vi "set ChildNode.vi"(8 "error in (no error)":errorcluster caption="错误输入（无错误）", 9 "ChildNode*":refnum<data-value>, 10 "index":i32 caption="L/R", 11 "PanelLinkNode输入":refnum<class "PanelLinkNode.lvclass">) -> (0 "error out":errorcluster caption="错误输出", 3 "PanelLinkNode输出":refnum<class "PanelLinkNode.lvclass">)   [LabVIEW 2016, in "PanelLinkNode.lvclass"]
uses:
  PanelLinkNode.lvclass
  PanelObject/PanelObject.lvclass
  PanelLinkNode.lvclass/PanelLinkNode.ctl
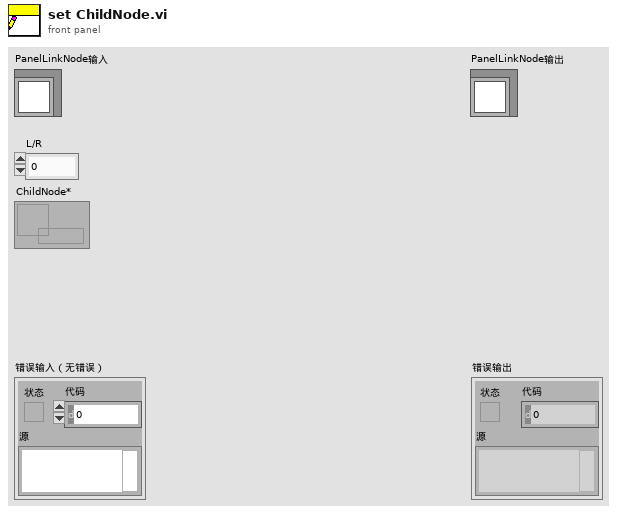
[diagram p1: front panel]
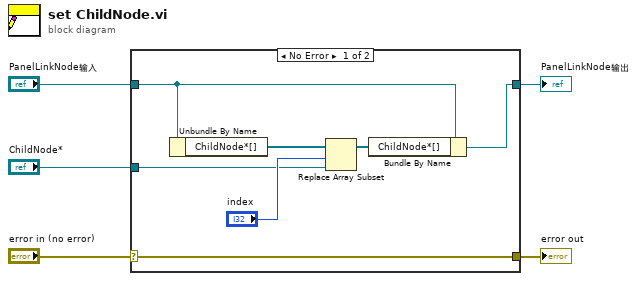
[diagram p0: block diagram]
diagram:
  n1 = case shown="No Error" "error in (no error)" {
    selector: "error in (no error)" -> [w12 w13]
    tunnel: [w12 w13] -> w4
    tunnel: [w11 w14] -> w2
    tunnel: "PanelLinkNode输入" -> [w10 w14]
    tunnel: "ChildNode*" -> [w6 _]
    frame No Error {
      n2 = Unbundle By Name(w10) -> ("ChildNode*[]"=w9:refnum<data-value>[])
      n3 = Replace Array Subset(array=w9, new element=w6, index="index") -> (w8:refnum<data-value>[])
      n4 = Bundle By Name(cluster=w10, "ChildNode*[]"=w8) -> (w11:refnum<class "PanelLinkNode.lvclass">)
    }
    frame Error {
    }
  }
  "error out" <- w4
  "PanelLinkNode输出" <- w2
